vi "Shutdown Daemon.vi"(8 "error in":errorcluster, 11 "TCP slave in":refnum<class "TCP Slave.lvclass">) -> (0 "error out":errorcluster)   [LabVIEW 2013, in "Modbus Library - Advance.lvlib" / "TCP Slave.lvclass"]
doc: "Sends a notification to the daemon and connection handlers, commanding them to quit."
uses:
  TCP Slave.lvclass
  Network Slave.lvclass
  TCP Slave.lvclass/TCP Slave.ctl
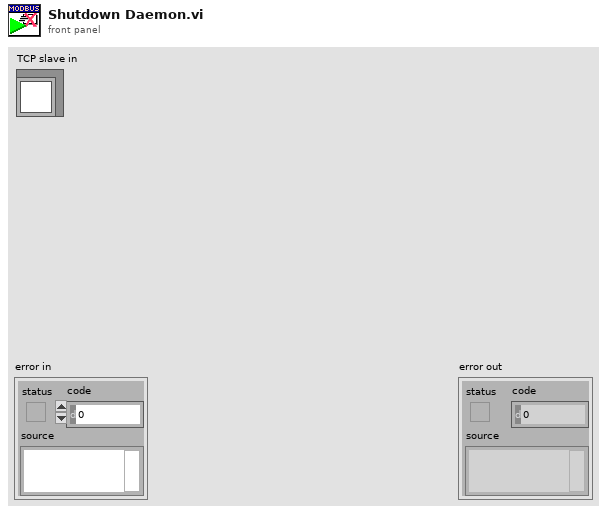
[diagram p1: front panel]
types:
  T1 = typedef "K2Labs Modbus Library.lvlib/TCP Slave.lvclass/Connection Counter.ctl" = cluster{"Currently Connected":u32, "Connection Records":refnum<data-value>[]}
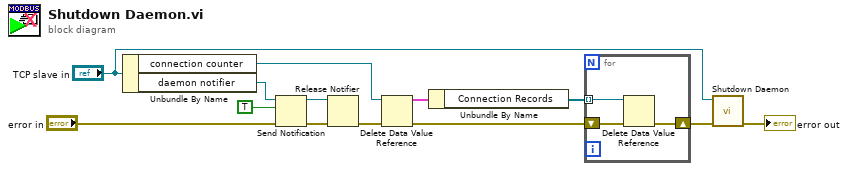
[diagram p0: block diagram]
diagram:
  n1 = Unbundle By Name("TCP slave in") -> ("connection counter"=w5:refnum<data-value>, "daemon notifier"=w10:refnum<notifier>)
  n2 = Send Notification(notification=TRUE, notifier=w10, error in (no error)="error in") -> (notifier out=w12:refnum<notifier>, error out=w11:errorcluster)
  n3 = Release Notifier(notifier=w12, error in (no error)=w11) -> (error out=w6:errorcluster)  [unwired: 1 in, 2 out]
  n4 = Delete Data Value Reference(data value reference=w5, error in=w6) -> (data value=w2:T1, error out=w4:errorcluster)
  n5 = Unbundle By Name(w2) -> ("Connection Records"=w1:refnum<data-value>[])
  n6 = for {
    shift-right: [w14] -> w3
    shift-left: w4 -> [w15]
    tunnel: w1 -> [w16] mode=indexing
    n7 = Delete Data Value Reference(data value reference=w16, error in=w15) -> (error out=w14:errorcluster)  [unwired: 1 out]
  }
  n8 = call-parent "Shutdown Daemon.vi"("error in"=w3, "network slave in"="TCP slave in") -> ("error out"=→"error out":errorcluster)  [unwired: 9 in]
